vi "Principal.vi"() -> ()   [LabVIEW 2020]
panel:
  in  "stop":bool
  in  "SEMAFORO":bool
  in  "DISPLAY":bool
  in  "LED":bool
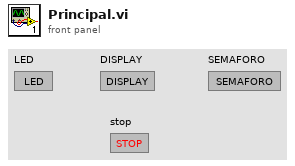
[diagram p1: front panel]
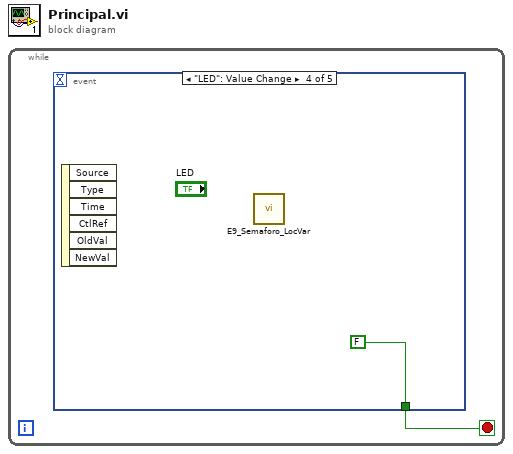
[diagram p0: block diagram]
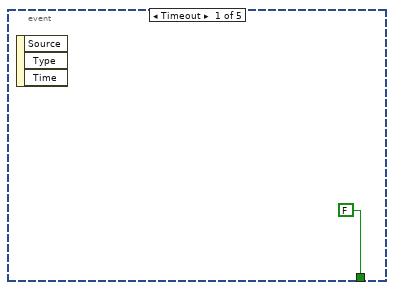
[diagram p2: hidden frame]
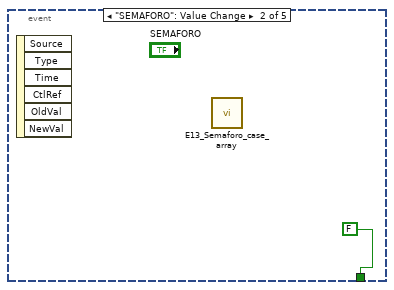
[diagram p3: hidden frame]
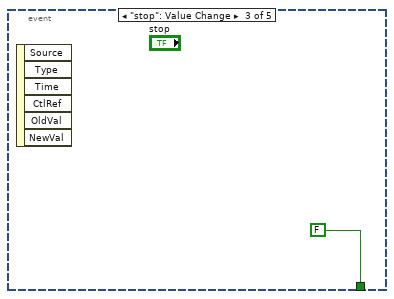
[diagram p4: hidden frame]
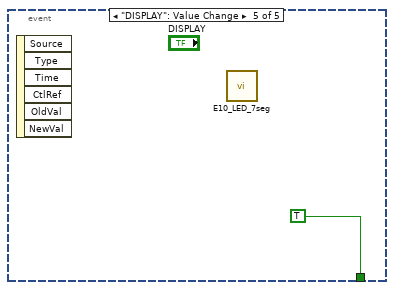
[diagram p5: hidden frame]
diagram:
  n1 = while {
    stop <- w1 stop-if-true
    n2 = event shown="[3] \"LED\": Value Change" {
      selector: _ -> [_ _ _ _ _]
      dyn-events: _ -> [_ _ _ _ _]
      timeout: _ -> [_ _ _ _ _]
      tunnel: [FALSE FALSE FALSE FALSE TRUE] -> w1
      event Timeout {
        n3 = event-data() -> ()  [unwired: 1 in, 3 out]
      }
      event "SEMAFORO": Value Change {
        n4 = event-data() -> ()  [unwired: 1 in, 6 out]
        n5 = call "E13_Semaforo_case_array.vi"() -> ()  [unwired: 12 out]
      }
      event "stop": Value Change {
        n6 = event-data() -> ()  [unwired: 1 in, 6 out]
      }
      event "LED": Value Change {
        n7 = event-data() -> ()  [unwired: 1 in, 6 out]
        n8 = call "E9_Semaforo_LocVar.vi"() -> ()  [unwired: 12 in]
      }
      event "DISPLAY": Value Change {
        n9 = event-data() -> ()  [unwired: 1 in, 6 out]
        n10 = call "E10_LED_7seg.vi"() -> ()  [unwired: 2 in, 7 out]
      }
    }
  }
